vi "GetCalibration.vi"(0 "VISA Refnum in":refnum<visa-resource-name>, 5 "error in (no error)":errorcluster) -> (10 "Temp (C)":sgl, 11 "OK result":bool, 12 "Tref":sgl[unit] format="%#_5g", 13 "Cycle time":dbl[unit], 14 "VISA Refnum out":refnum<visa-resource-name>, 15 "Clock factor":u8, 16 "Res. Theor. cycles":sgl, 17 "Res. cycles":sgl, 18 "TDC cycles":u16, 19 "error out":errorcluster)   [LabVIEW 2013]
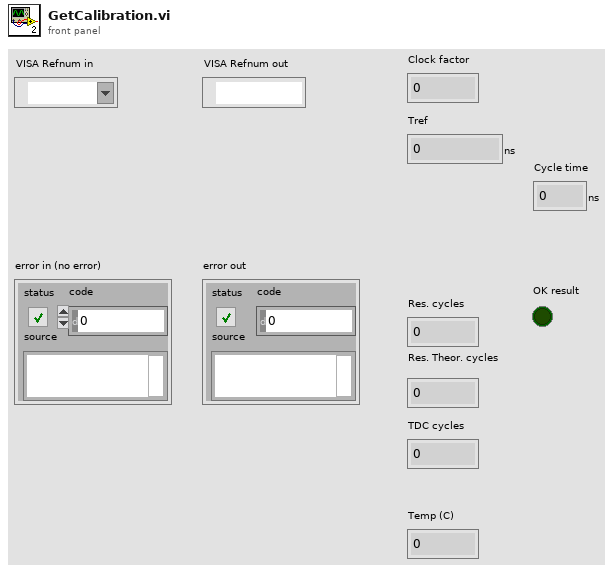
[diagram p1: front panel]
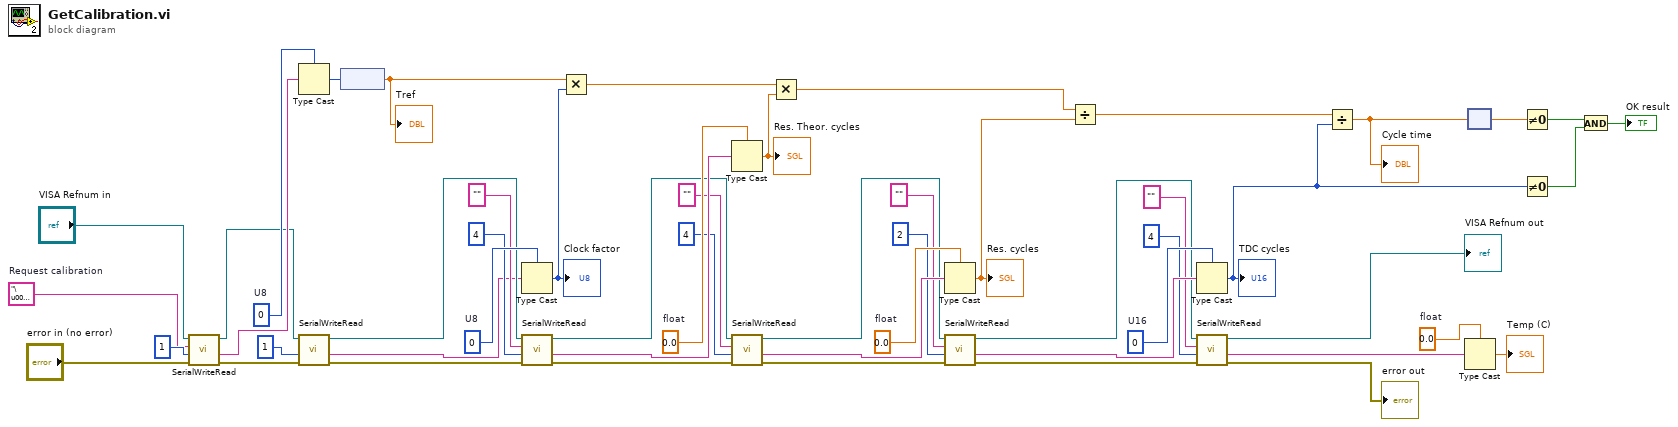
[diagram p0: block diagram]
diagram:
  w2 = sgl 0.0  # float
  w30 = u16 0  # U16
  w36 = sgl 0.0  # float
  w42 = sgl 0.0  # float
  w43 = u8 0  # U8
  w48 = "\u0003"  # Request calibration
  w47 = u8 0  # U8
  n1 = call "SerialWriteRead.vi"("error in (no error)"="error in (no error)", "Bytes to read"=u32 1 ("byte count"), "The byte to send before reading"=w48, "VISA Refnum in"="VISA Refnum in") -> ("error out"=w45:errorcluster, "Hex Out"=w52:string, "VISA Refnum out"=w44:refnum<visa-resource-name>)  [unwired: 4 in, 1 out]
  n2 = Type Cast(type=w47, x=w52) -> (*(type *) &x=w46:u8)
  n3 = call "SerialWriteRead.vi"("error in (no error)"=w45, "Bytes to read"=u32 1 ("byte count"), "VISA Refnum in"=w44) -> ("error out"=w40:errorcluster, "Hex Out"=w23:string, "VISA Refnum out"=w41:refnum<visa-resource-name>)  [unwired: 5 in, 1 out]
  n4 = node(w46) -> (w22:dbl[unit])
  "Tref" <- w22
  n5 = Type Cast(type=w43, x=w23) -> (*(type *) &x=w21:u8)
  "Clock factor" <- w21
  n6 = call "SerialWriteRead.vi"("error in (no error)"=w40, "Bytes to read"=u32 4 ("byte count"), "The byte to send before reading"="" ("Opcode"), "VISA Refnum in"=w41) -> ("error out"=w31:errorcluster, "Hex Out"=w37:string, "VISA Refnum out"=w32:refnum<visa-resource-name>)  [unwired: 4 in, 1 out]
  n7 = Multiply(x=w22, y=w21) -> (x*y=w20:dbl[unit])
  n8 = Type Cast(type=w42, x=w37) -> (*(type *) &x=w19:sgl)
  "Res. Theor. cycles" <- w19
  n9 = call "SerialWriteRead.vi"("error in (no error)"=w31, "Bytes to read"=u32 4 ("byte count"), "The byte to send before reading"="" ("Opcode"), "VISA Refnum in"=w32) -> ("error out"=w25:errorcluster, "Hex Out"=w33:string, "VISA Refnum out"=w26:refnum<visa-resource-name>)  [unwired: 4 in, 1 out]
  n10 = Multiply(x=w20, y=w19) -> (x*y=w18:dbl[unit])
  n11 = Type Cast(type=w36, x=w33) -> (*(type *) &x=w17:sgl)
  "Res. cycles" <- w17
  n12 = call "SerialWriteRead.vi"("error in (no error)"=w25, "Bytes to read"=u32 2 ("byte count"), "The byte to send before reading"="" ("Opcode"), "VISA Refnum in"=w26) -> ("error out"=w5:errorcluster, "Hex Out"=w27:string, "VISA Refnum out"=w9:refnum<visa-resource-name>)  [unwired: 4 in, 1 out]
  n13 = Divide(x=w18, y=w17) -> (x/y=w16:dbl[unit])
  n14 = Type Cast(type=w30, x=w27) -> (*(type *) &x=w15:u16)
  "TDC cycles" <- w15
  n15 = call "SerialWriteRead.vi"("error in (no error)"=w5, "Bytes to read"=u32 4 ("byte count"), "The byte to send before reading"="" ("Opcode"), "VISA Refnum in"=w9) -> ("error out"=→"error out":errorcluster, "Hex Out"=w3:string, "VISA Refnum out"=→"VISA Refnum out":refnum<visa-resource-name>)  [unwired: 4 in, 1 out]
  n16 = Divide(x=w16, y=w15) -> (x/y=w14:dbl[unit])
  "Cycle time" <- w14
  n17 = Type Cast(type=w2, x=w3) -> (*(type *) &x=→"Temp (C)":sgl)
  n18 = node(w14) -> (w13:dbl)
  n19 = Not Equal To 0?(x=w13) -> (x != 0?=w11:bool)
  n20 = Not Equal To 0?(x=w15) -> (x != 0?=w12:bool)
  n21 = And(x=w11, y=w12) -> (x .and. y?=→"OK result":bool)
